vi "main-sequential.vi"() -> ()   [LabVIEW 2024]
uses:
  controls/thermocouple-input-cluster.ctl
  controls/analog-input-cluster.ctl
  controls/analog-output-cluster.ctl
  controls/digitial-input-cluster.ctl
  controls/digital-output-cluster.ctl
  controls/adam-module-select-tab.ctl
  controls/adam-5000-serial-settings.ctl
  controls/state-enum.ctl
  controls/adam-5000-all-chassis-data.ctl
  controls/adam-5000-all-module-datas.ctl
  controls/adam-5000-chassis-cmd-ack.ctl
  controls/adam-5000-module-cmd-ack.ctl
  <vilib>/Instr/_visa.llb/VISA Configure Serial Port (Instr).vi
  <vilib>/Instr/_visa.llb/VISA Flush IO Buffer Mask.ctl
panel:
  out "response":string
  out "cmd string":string
  out "Ack":bool
  out "Sampling":bool
  in  "Slot 1: Module Type":T1(ring)=enum."Thermocouple"
  out "slot: 1":T2
  in  "Digital Outputs 2":T3
  out "Digital Inputs 2":T4
  in  "Analog Outputs 2":T5
  out "Analog Inputs 2":T6
  out "Thermocouple Inputs (degC) 2":T7
  out "response":string
  out "cmd string":string
  out "Ack":bool
  out "Sampling":bool
  in  "Slot 0: Module Type":T1(ring)=enum."Analog Input"
  out "slot: 0":T2
  in  "Digital Outputs":T3
  out "Digital Inputs":T4
  in  "Analog Outputs":T5
  out "Analog Inputs":T6
  out "Thermocouple Inputs (degC)":T7
  in  "Chassis Settings":T8={"VISA resource name"="COM10", "baud rate (19200)"=19200, "Chassis ID"=1}
  in  "Debug Mode":bool
  out "Loop Time (mS)":u32
  out "Loop Counter":i32
  out "Write Success":bool
  out "error IO":errorcluster
  out "error":errorcluster
  in  "exit":bool
  # "ADAM 5000 Controller"
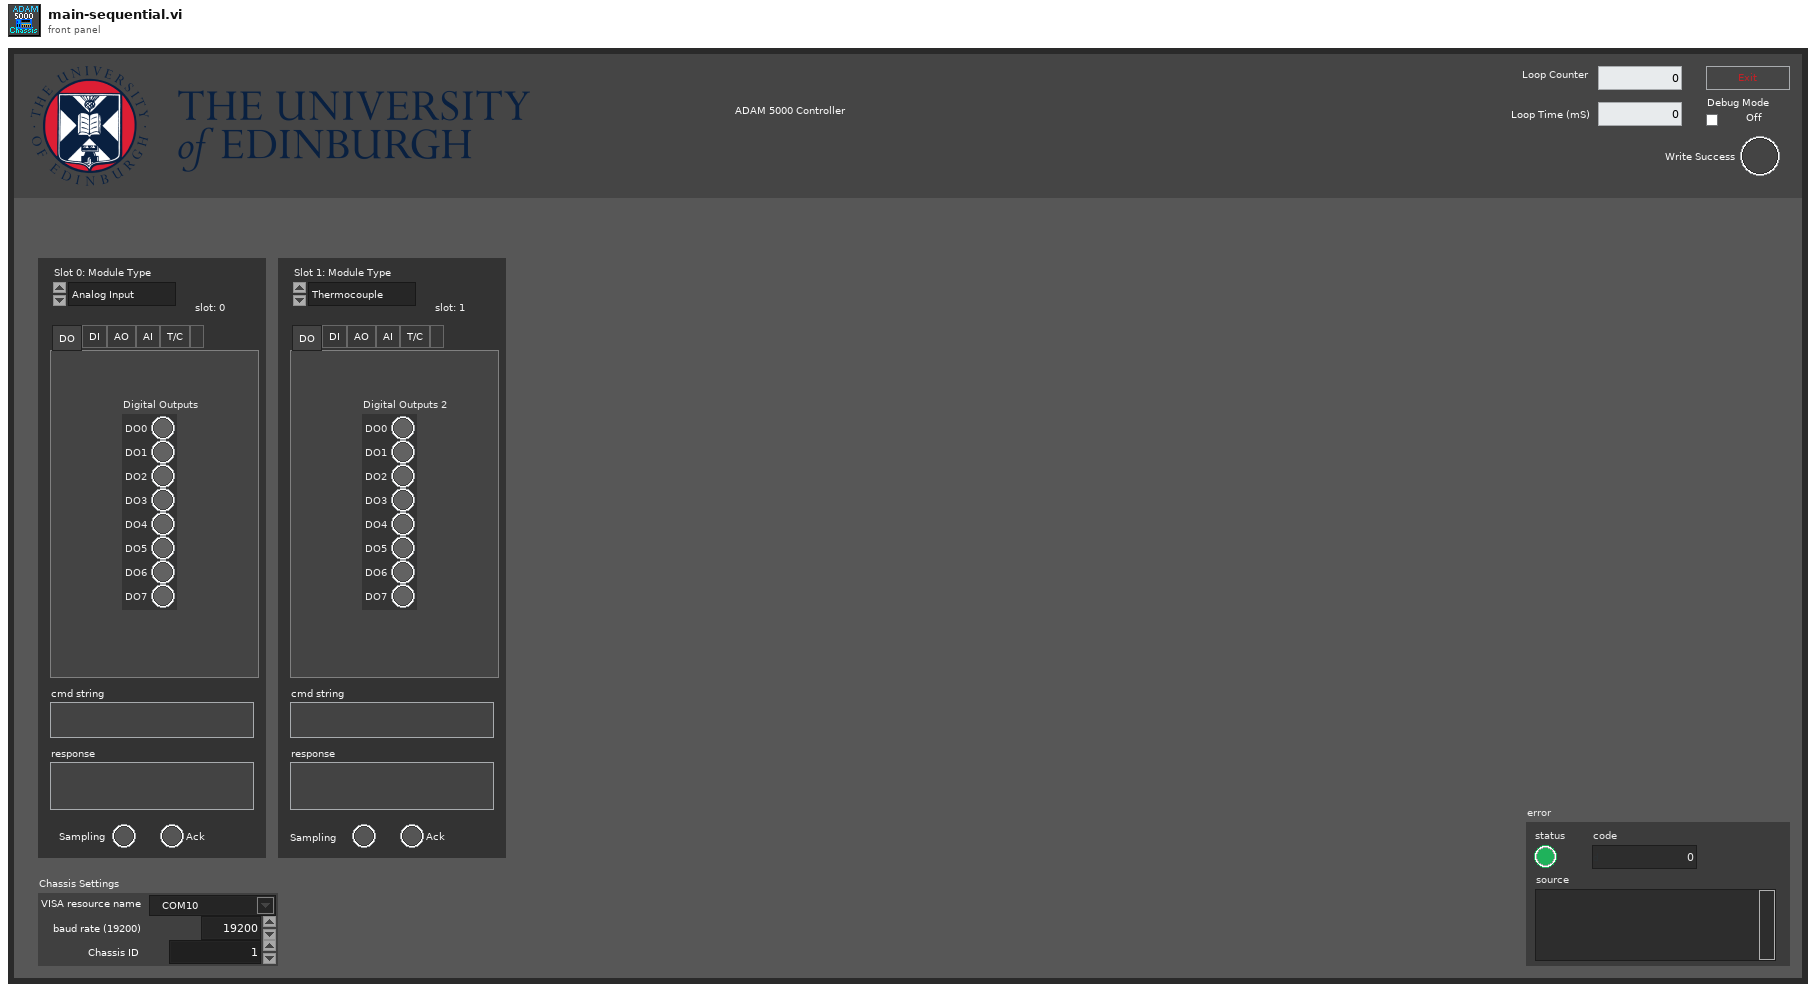
[diagram p1: front panel]
types:
  T1 = enum16{"Digital Output", "Digital Input", "Analog Output", "Analog Input", "Thermocouple", "Power Relay", "empty"}
  T2 = typedef "adam-module-select-tab.ctl" = enum32{"DO", "DI", "AO", "AI", "T/C", ""}
  T3 = typedef "digital-output-cluster.ctl" = cluster{"DO0":bool, "DO1":bool, "DO2":bool, "DO3":bool, "DO4":bool, "DO5":bool, "DO6":bool, "DO7":bool}
  T4 = typedef "digitial-input-cluster.ctl" = cluster{"DI0":bool, "DI1":bool, "DI2":bool, "DI3":bool, "DI4":bool, "DI5":bool, "DI6":bool, "DI7":bool}
  T5 = typedef "analog-output-cluster.ctl" = cluster{"AO0":dbl, "AO1":dbl, "AO2":dbl, "AO3":dbl}
  T6 = typedef "analog-input-cluster.ctl" = cluster{"AI0":dbl, "AI1":dbl, "AI2":dbl, "AI3":dbl, "AI4":dbl, "AI5":dbl, "AI6":dbl, "AI7":dbl}
  T7 = typedef "thermocouple-input-cluster.ctl" = cluster{"TC0":dbl, "TC1":dbl, "TC2":dbl, "TC3":dbl, "TC4":dbl, "TC5":dbl, "TC6":dbl}
  T8 = typedef "adam-5000-serial-settings.ctl" = cluster{"VISA resource name":refnum<visa-resource-name>, "baud rate (19200)":u32, "Chassis ID":u8}
  T9 = typedef "adam-5000-chassis-cmd-ack.ctl" = cluster{"0 cmd-ack":T10, "1 cmd-ack":T10, "2 cmd-ack":T10, "3 cmd-ack":T10, "4 cmd-ack":T10, "5 cmd-ack":T10, "6 cmd-ack":T10, "7 cmd-ack":T10}
  T10 = typedef "adam-5000-module-cmd-ack.ctl" = cluster{"cmd out":string, "acknowledge char":string}
  T11 = typedef "adam-5000-all-chassis-data.ctl" = cluster{"slot:0":T12, "slot:1":T12, "slot:2":T12, "slot:3":T12, "slot:4":T12, "slot:5":T12, "slot:6":T12, "slot:7":T12}
  T12 = typedef "adam-5000-all-module-datas.ctl" = cluster{"Digital Outputs":T3, "Digital Inputs":T4, "Analog Outputs":T5, "Analog Inputs":T6, "Thermocouple Inputs (degC)":T7}
  T13 = typedef "state-enum.ctl" = enum16{"init", "manual", "start", "run", "hold", "stop", ""}
  T14 = cluster{"Analog Outputs":T5, "Analog Outputs 2":T5}
  T15 = cluster{"Slot 0: Module Type":enum16{"Digital Output", "Digital Input", "Analog Output", "Analog Input", "Thermocouple", "Power Relay", "empty"}, "Slot 1: Module Type":enum16{"Digital Output", "Digital Input", "Analog Output", "Analog Input", "Thermocouple", "Power Relay", "empty"}}
  T16 = cluster{"Digital Outputs":T3, "Digital Outputs 2":T3}
  T17 = cluster{"[0]":T10, "[1]":T10, "[2]":T10, "[3]":T10, "[4]":T10, "[5]":T10, "[6]":T10, "[7]":T10, "[8]":T10}
  T18 = typedef "VISA Flush IO Buffer Mask.ctl" = u16
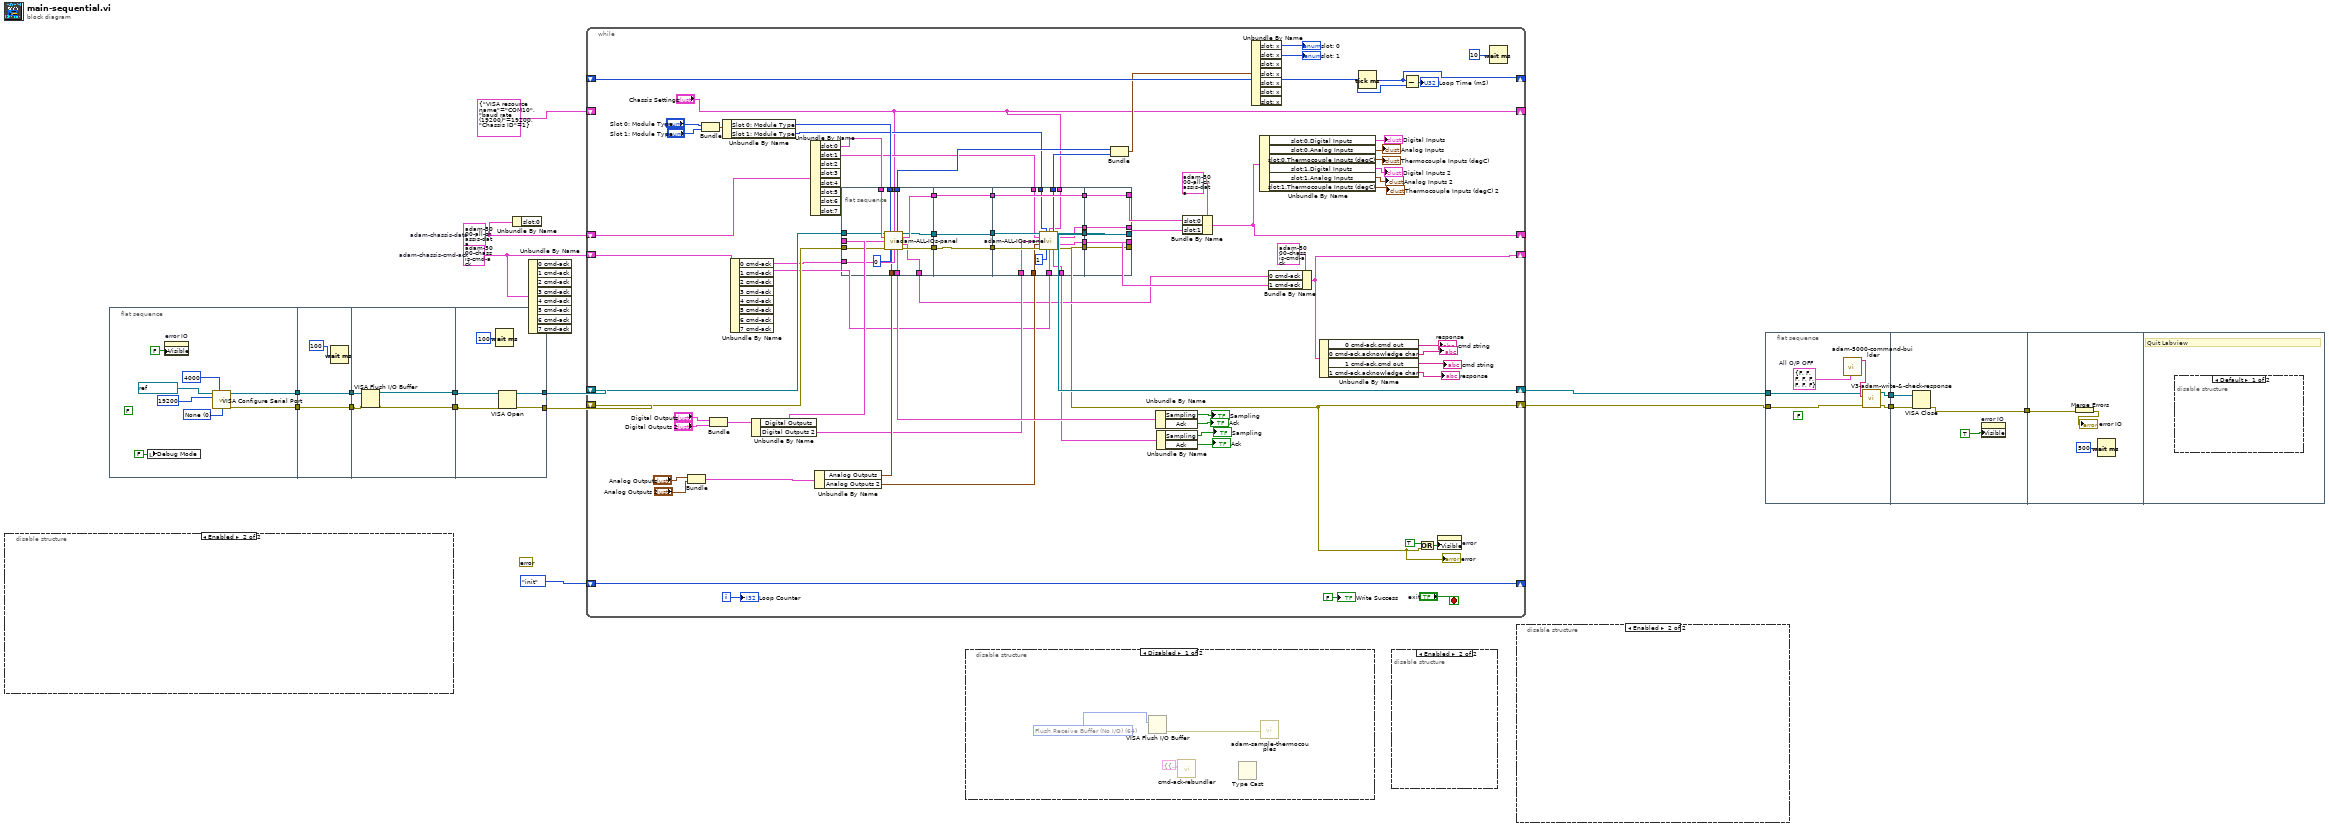
[diagram p0: block diagram]
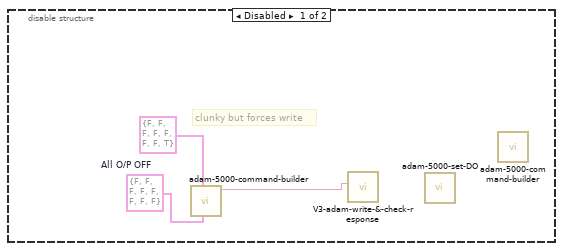
[diagram p2: hidden frame]
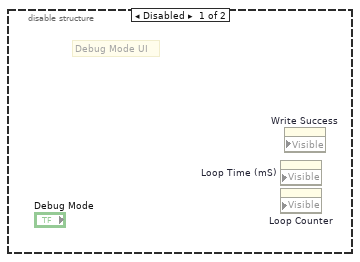
[diagram p3: hidden frame]
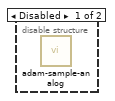
[diagram p4: hidden frame]
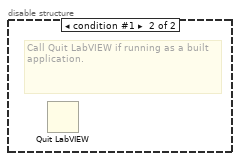
[diagram p6: hidden frame]
diagram:
  w1 = T9 {"0 cmd-ack"={"cmd out"="", "acknowledge char"=""}, "1 cmd-ack"={"cmd out"="", "acknowledge char"=""}, "2 cmd-ack"={"cmd out"="", "acknowledge char"=""}, "3 cmd-ack"={"cmd out"="", "acknowledge char"=""}, "4 cmd-ack"={"cmd out"="", "acknowledge char"=""}, "5 cmd-ack"={"cmd out"="", "acknowledge char"=""}, "6 cmd-ack"={"cmd out"="", "acknowledge char"=""}, "7 cmd-ack"={"cmd out"="", "acknowledge char"=""}}  # adam-chassis-cmd-ack
  w2 = T11 {"slot:0"={"Digital Outputs"={"DO0"=FALSE, "DO1"=FALSE, "DO2"=FALSE, "DO3"=FALSE, "DO4"=FALSE, "DO5"=FALSE, "DO6"=FALSE, "DO7"=FALSE}, "Digital Inputs"={"DI0"=FALSE, "DI1"=FALSE, "DI2"=FALSE, "DI3"=FALSE, "DI4"=FALSE, "DI5"=FALSE, "DI6"=FALSE, "DI7"=FALSE}, "Analog Outputs"={"AO0"=0.0, "AO1"=0.0, "AO2"=0.0, "AO3"=0.0}, "Analog Inputs"={"AI0"=0.0, "AI1"=0.0, "AI2"=0.0, "AI3"=0.0, "AI4"=0.0, "AI5"=0.0, "AI6"=0.0, "AI7"=0.0}, "Thermocouple Inputs (degC)"={"TC0"=0.0, "TC1"=0.0, "TC2"=0.0, "TC3"=0.0, "TC4"=0.0, "TC5"=0.0, "TC6"=0.0}}, "slot:1"={"Digital Outputs"={"DO0"=FALSE, "DO1"=FALSE, "DO2"=FALSE, "DO3"=FALSE, "DO4"=FALSE, "DO5"=FALSE, "DO6"=FALSE, "DO7"=FALSE}, "Digital Inputs"={"DI0"=FALSE, "DI1"=FALSE, "DI2"=FALSE, "DI3"=FALSE, "DI4"=FALSE, "DI5"=FALSE, "DI6"=FALSE, "DI7"=FALSE}, "Analog Outputs"={"AO0"=0.0, "AO1"=0.0, "AO2"=0.0, "AO3"=0.0}, "Analog Inputs"={"AI0"=0.0, "AI1"=0.0, "AI2"=0.0, "AI3"=0.0, "AI4"=0.0, "AI5"=0.0, "AI6"=0.0, "AI7"=0.0}, "Thermocouple Inputs (degC)"={"TC0"=0.0, "TC1"=0.0, "TC2"=0.0, "TC3"=0.0, "TC4"=0.0, "TC5"=0.0, "TC6"=0.0}}, "slot:2"={"Digital Outputs"={"DO0"=FALSE, "DO1"=FALSE, "DO2"=FALSE, "DO3"=FALSE, "DO4"=FALSE, "DO5"=FALSE, "DO6"=FALSE, "DO7"=FALSE}, "Digital Inputs"={"DI0"=FALSE, "DI1"=FALSE, "DI2"=FALSE, "DI3"=FALSE, "DI4"=FALSE, "DI5"=FALSE, "DI6"=FALSE, "DI7"=FALSE}, "Analog Outputs"={"AO0"=0.0, "AO1"=0.0, "AO2"=0.0, "AO3"=0.0}, "Analog Inputs"={"AI0"=0.0, "AI1"=0.0, "AI2"=0.0, "AI3"=0.0, "AI4"=0.0, "AI5"=0.0, "AI6"=0.0, "AI7"=0.0}, "Thermocouple Inputs (degC)"={"TC0"=0.0, "TC1"=0.0, "TC2"=0.0, "TC3"=0.0, "TC4"=0.0, "TC5"=0.0, "TC6"=0.0}}, "slot:3"={"Digital Outputs"={"DO0"=FALSE, "DO1"=FALSE, "DO2"=FALSE, "DO3"=FALSE, "DO4"=FALSE, "DO5"=FALSE, "DO6"=FALSE, "DO7"=FALSE}, "Digital Inputs"={"DI0"=FALSE, "DI1"=FALSE, "DI2"=FALSE, "DI3"=FALSE, "DI4"=FALSE, "DI5"=FALSE, "DI6"=FALSE, "DI7"=FALSE}, "Analog Outputs"={"AO0"=0.0, "AO1"=0.0, "AO2"=0.0, "AO3"=0.0}, "Analog Inputs"={"AI0"=0.0, "AI1"=0.0, "AI2"=0.0, "AI3"=0.0, "AI4"=0.0, "AI5"=0.0, "AI6"=0.0, "AI7"=0.0}, "Thermocouple Inputs (degC)"={"TC0"=0.0, "TC1"=0.0, "TC2"=0.0, "TC3"=0.0, "TC4"=0.0, "TC5"=0.0, "TC6"=0.0}}, "slot:4"={"Digital Outputs"={"DO0"=FALSE, "DO1"=FALSE, "DO2"=FALSE, "DO3"=FALSE, "DO4"=FALSE, "DO5"=FALSE, "DO6"=FALSE, "DO7"=FALSE}, "Digital Inputs"={"DI0"=FALSE, "DI1"=FALSE, "DI2"=FALSE, "DI3"=FALSE, "DI4"=FALSE, "DI5"=FALSE, "DI6"=FALSE, "DI7"=FALSE}, "Analog Outputs"={"AO0"=0.0, "AO1"=0.0, "AO2"=0.0, "AO3"=0.0}, "Analog Inputs"={"AI0"=0.0, "AI1"=0.0, "AI2"=0.0, "AI3"=0.0, "AI4"=0.0, "AI5"=0.0, "AI6"=0.0, "AI7"=0.0}, "Thermocouple Inputs (degC)"={"TC0"=0.0, "TC1"=0.0, "TC2"=0.0, "TC3"=0.0, "TC4"=0.0, "TC5"=0.0, "TC6"=0.0}}, "slot:5"={"Digital Outputs"={"DO0"=FALSE, "DO1"=FALSE, "DO2"=FALSE, "DO3"=FALSE, "DO4"=FALSE, "DO5"=FALSE, "DO6"=FALSE, "DO7"=FALSE}, "Digital Inputs"={"DI0"=FALSE, "DI1"=FALSE, "DI2"=FALSE, "DI3"=FALSE, "DI4"=FALSE, "DI5"=FALSE, "DI6"=FALSE, "DI7"=FALSE}, "Analog Outputs"={"AO0"=0.0, "AO1"=0.0, "AO2"=0.0, "AO3"=0.0}, "Analog Inputs"={"AI0"=0.0, "AI1"=0.0, "AI2"=0.0, "AI3"=0.0, "AI4"=0.0, "AI5"=0.0, "AI6"=0.0, "AI7"=0.0}, "Thermocouple Inputs (degC)"={"TC0"=0.0, "TC1"=0.0, "TC2"=0.0, "TC3"=0.0, "TC4"=0.0, "TC5"=0.0, "TC6"=0.0}}, "slot:6"={"Digital Outputs"={"DO0"=FALSE, "DO1"=FALSE, "DO2"=FALSE, "DO3"=FALSE, "DO4"=FALSE, "DO5"=FALSE, "DO6"=FALSE, "DO7"=FALSE}, "Digital Inputs"={"DI0"=FALSE, "DI1"=FALSE, "DI2"=FALSE, "DI3"=FALSE, "DI4"=FALSE, "DI5"=FALSE, "DI6"=FALSE, "DI7"=FALSE}, "Analog Outputs"={"AO0"=0.0, "AO1"=0.0, "AO2"=0.0, "AO3"=0.0}, "Analog Inputs"={"AI0"=0.0, "AI1"=0.0, "AI2"=0.0, "AI3"=0.0, "AI4"=0.0, "AI5"=0.0, "AI6"=0.0, "AI7"=0.0}, "Thermocouple Inputs (degC)"={"TC0"=0.0, "TC1"=0.0, "TC2"=0.0, "TC3"=0.0, "TC4"=0.0, "TC5"=0.0, "TC6"=0.0}}, "slot:7"={"Digital Outputs"={"DO0"=FALSE, "DO1"=FALSE, "DO2"=FALSE, "DO3"=FALSE, "DO4"=FALSE, "DO5"=FALSE, "DO6"=FALSE, "DO7"=FALSE}, "Digital Inputs"={"DI0"=FALSE, "DI1"=FALSE, "DI2"=FALSE, "DI3"=FALSE, "DI4"=FALSE, "DI5"=FALSE, "DI6"=FALSE, "DI7"=FALSE}, "Analog Outputs"={"AO0"=0.0, "AO1"=0.0, "AO2"=0.0, "AO3"=0.0}, "Analog Inputs"={"AI0"=0.0, "AI1"=0.0, "AI2"=0.0, "AI3"=0.0, "AI4"=0.0, "AI5"=0.0, "AI6"=0.0, "AI7"=0.0}, "Thermocouple Inputs (degC)"={"TC0"=0.0, "TC1"=0.0, "TC2"=0.0, "TC3"=0.0, "TC4"=0.0, "TC5"=0.0, "TC6"=0.0}}}  # adam-chassis-data
  (unwired) errorcluster {"status"=FALSE, "code"=0, "source"=""} ("error")
  n1 = disable-structure shown="Enabled" {
    frame Disabled {
      w20 = T3 {"DO0"=FALSE, "DO1"=FALSE, "DO2"=FALSE, "DO3"=FALSE, "DO4"=FALSE, "DO5"=FALSE, "DO6"=FALSE, "DO7"=FALSE}  # All O/P OFF
      # "clunky but forces write"
      n2 = call "adam-5000-command-builder.vi"("Output Control"=w20, "Current Output State"=T3 {"DO0"=FALSE, "DO1"=FALSE, "DO2"=FALSE, "DO3"=FALSE, "DO4"=FALSE, "DO5"=FALSE, "DO6"=FALSE, "DO7"=TRUE}) -> ("Command Out"=w19:string)  [unwired: 7 in, 2 out]
      n3 = call "V3-adam-write-&-check-response.vi"("write buffer"=w19) -> ("VISA resource name"=w18:refnum<visa-resource-name>)  [unwired: 5 in, 5 out]
      n4 = call "adam-5000-set-DO.vi"() -> ()  [unwired: 6 in, 6 out]
      n5 = call "adam-5000-command-builder.vi"() -> ()  [unwired: 9 in, 3 out]
    }
    frame Enabled {
    }
  }
  n6 = flat-sequence {
    tunnel: [w28] -> w11
    tunnel: [w27] -> w10
    tunnel: w11 -> [w32]
    tunnel: [w32] -> w9
    tunnel: w10 -> [w31]
    tunnel: [w31] -> w8
    tunnel: w9 -> [w36]
    tunnel: [w34] -> w7
    tunnel: w8 -> [w35]
    tunnel: [w33] -> w6
    tunnel: w7 -> [w40]
    tunnel: w6 -> [w39]
    tunnel: [w38] -> w5
    tunnel: [w37] -> w4
    frame #0 {
      w25 = u16 0 items=["None", "XON/XOFF", "RTS/CTS", "XON/XOFF & RTS/CTS", "DTR/DSR", "XON/XOFF & DTR/DSR"] ("flow control (0:none)")
      (unwired) FALSE ("V1")
      n7 = local write "Debug Mode"(FALSE ("Debug Mode")) -> ()
      n8 = property on="error IO" class="Clust (strict)"("Visible"=FALSE) -> ()  [unwired: 2 in, 2 out]
      n9 = call-poly "VISA Configure Serial Port"("VISA resource name"=refnum<visa-resource-name> "COM10", "timeout (10sec)"=u32 4000, "baud rate (9600)"=u32 19200, "flow control (0:none)"=w25) -> ("VISA resource name out"=w28:refnum<visa-resource-name>, "error out"=w27:errorcluster)  [unwired: 10 in]
    }
    frame #1 {
      n10 = Wait (ms)(milliseconds to wait=u32 100) -> ()  [unwired: 1 out]
    }
    frame #2 {
      n11 = VISA Flush I/O Buffer(VISA resource name=w36, error in (no error)=w35) -> (VISA resource name out=w34:refnum<visa-resource-name>, error out=w33:errorcluster)  [unwired: 1 in]
    }
    frame #3 {
      n12 = Wait (ms)(milliseconds to wait=u32 100) -> ()  [unwired: 1 out]
      n13 = VISA Open(error in (no error)=w39, VISA resource name=w40) -> (VISA resource name=w38:refnum<visa-resource-name>, error out=w37:errorcluster)  [unwired: 3 in]
    }
  }
  n14 = Unbundle By Name(w2) -> ()  [unwired: 1 out]
  n15 = Unbundle By Name(w1) -> ()  [unwired: 8 out]
  n16 = while {
    shift-right: [w109] -> _
    shift-left: state-enum."init" ("state-enum") -> [w109]
    shift-right: [w48] -> w16
    shift-left: w4 -> [w90]
    shift-right: [w112] -> _
    shift-left: _ -> [w114]
    shift-right: ["Chassis Settings"] -> _
    shift-left: T8 {"VISA resource name"="COM10", "baud rate (19200)"=19200, "Chassis ID"=1} ("Chassis Settings") -> [_]
    shift-right: [w69] -> w3
    shift-left: w5 -> [w91]
    shift-right: [w74] -> _
    shift-left: w2 -> [w42]
    shift-right: [w85] -> _
    shift-left: w1 -> [w93]
    i -> [w115]
    stop <- "exit" stop-if-true
    n17 = Bundle("Analog Outputs"="Analog Outputs", "Analog Outputs 2"="Analog Outputs 2") -> (w82:T14)  [unwired: 1 in]
    n18 = Bundle("Slot 0: Module Type"="Slot 0: Module Type", "Slot 1: Module Type"="Slot 1: Module Type") -> (w80:T15)  [unwired: 1 in]
    n19 = Bundle("Digital Outputs"="Digital Outputs", "Digital Outputs 2"="Digital Outputs 2") -> (w84:T16)  [unwired: 1 in]
    n20 = Unbundle By Name(w80) -> ("Slot 0: Module Type"=w79:T1, "Slot 1: Module Type"=w59:T1)
    n21 = Unbundle By Name(w93) -> ("0 cmd-ack"=w89:T10, "1 cmd-ack"=w61:T10)  [unwired: 6 out]
    n22 = Unbundle By Name(w84) -> ("Digital Outputs"=w83:T3, "Digital Outputs 2"=w63:T3)
    n23 = Unbundle By Name(w42) -> ("slot:0"=w92:T12, "slot:1"=w65:T12)  [unwired: 6 out]
    n24 = Unbundle By Name(w82) -> ("Analog Outputs"=w81:T5, "Analog Outputs 2"=w62:T5)
    n25 = flat-sequence {
      tunnel: w92 -> [w132]
      tunnel: w91 -> [w131]
      tunnel: w90 -> [w130]
      tunnel: w89 -> [w129]
      tunnel: w83 -> [w127]
      tunnel: w81 -> [w126]
      tunnel: "Chassis Settings" -> [w125]
      tunnel: w79 -> [w124]
      tunnel: [w123] -> w78
      tunnel: [w121] -> w68
      tunnel: [w128] -> w55
      tunnel: [w122] -> w53
      tunnel: [w119] -> w51
      tunnel: [w118] -> w49
      tunnel: w55 -> [w135]
      tunnel: [w135] -> w54
      tunnel: w53 -> [w134]
      tunnel: [w134] -> w52
      tunnel: w51 -> [w133]
      tunnel: [w133] -> w50
      tunnel: w54 -> [w151]
      tunnel: w52 -> [w150]
      tunnel: w50 -> [w148]
      tunnel: w65 -> [w146]
      tunnel: w63 -> [w144]
      tunnel: w62 -> [w143]
      tunnel: w61 -> [w141]
      tunnel: w59 -> [w139]
      tunnel: [w138] -> w58
      tunnel: "Chassis Settings" -> [w137]
      tunnel: [w136] -> w56
      tunnel: [w151] -> w47
      tunnel: [w149] -> w46
      tunnel: [w147] -> w45
      tunnel: [w145] -> w44
      tunnel: [w140] -> w43
      tunnel: [w152] -> w60
      tunnel: [w153] -> w64
      tunnel: [w154] -> w48
      tunnel: [w155] -> w69
      tunnel: [w156] -> w87
      tunnel: w47 -> [w156]
      tunnel: w46 -> [w155]
      tunnel: w45 -> [w154]
      tunnel: w44 -> [w153]
      tunnel: w43 -> [w152]
      frame #0 {
        n26 = call "adam-ALL-IOs-panel.vi"("VISA Refnum in"=w131, "Module Type"=w124, "Chassis Settings"=w125, "ADAM-5000-data-current"=w132, "Digital Outputs"=w127, "Analog Outputs"=w126, "error in (no error)"=w130, "chassis-slot"=0, "cmd-ack-in"=w129) -> ("slot: x"=w123:T2, "VISA Refnum out"=w122:refnum<visa-resource-name>, "ADAM-5000-data-new"=w128:T12, "cmd-ack-out"=w118:T10, "status-cluster"=w121:cluster{"Sampling":bool, "Ack":bool}, "error out"=w119:errorcluster)  [unwired: 1 in]
      }
      frame #1 {
      }
      frame #2 {
        n27 = call "adam-ALL-IOs-panel.vi"("VISA Refnum in"=w150, "Module Type"=w139, "Chassis Settings"=w137, "ADAM-5000-data-current"=w146, "Digital Outputs"=w144, "Analog Outputs"=w143, "error in (no error)"=w148, "chassis-slot"=1, "cmd-ack-in"=w141) -> ("slot: x"=w138:T2, "VISA Refnum out"=w149:refnum<visa-resource-name>, "ADAM-5000-data-new"=w145:T12, "cmd-ack-out"=w140:T10, "status-cluster"=w136:cluster{"Sampling":bool, "Ack":bool}, "error out"=w147:errorcluster)  [unwired: 1 in]
      }
      frame #3 {
      }
    }
    n28 = Bundle("slot: x"=w78, "slot: x"=w58) -> (w77:cluster{"slot: x":T2, "slot: x":T2})  [unwired: 1 in]
    n29 = Unbundle By Name(w68) -> ("Sampling"=→"Sampling":bool, "Ack"=→"Ack":bool)
    n30 = Unbundle By Name(w56) -> ("Sampling"=→"Sampling":bool, "Ack"=→"Ack":bool)
    n31 = Bundle By Name(cluster=T11 {"slot:0"={"Digital Outputs"={"DO0"=FALSE, "DO1"=FALSE, "DO2"=FALSE, "DO3"=FALSE, "DO4"=FALSE, "DO5"=FALSE, "DO6"=FALSE, "DO7"=FALSE}, "Digital Inputs"={"DI0"=FALSE, "DI1"=FALSE, "DI2"=FALSE, "DI3"=FALSE, "DI4"=FALSE, "DI5"=FALSE, "DI6"=FALSE, "DI7"=FALSE}, "Analog Outputs"={"AO0"=0.0, "AO1"=0.0, "AO2"=0.0, "AO3"=0.0}, "Analog Inputs"={"AI0"=0.0, "AI1"=0.0, "AI2"=0.0, "AI3"=0.0, "AI4"=0.0, "AI5"=0.0, "AI6"=0.0, "AI7"=0.0}, "Thermocouple Inputs (degC)"={"TC0"=0.0, "TC1"=0.0, "TC2"=0.0, "TC3"=0.0, "TC4"=0.0, "TC5"=0.0, "TC6"=0.0}}, "slot:1"={"Digital Outputs"={"DO0"=FALSE, "DO1"=FALSE, "DO2"=FALSE, "DO3"=FALSE, "DO4"=FALSE, "DO5"=FALSE, "DO6"=FALSE, "DO7"=FALSE}, "Digital Inputs"={"DI0"=FALSE, "DI1"=FALSE, "DI2"=FALSE, "DI3"=FALSE, "DI4"=FALSE, "DI5"=FALSE, "DI6"=FALSE, "DI7"=FALSE}, "Analog Outputs"={"AO0"=0.0, "AO1"=0.0, "AO2"=0.0, "AO3"=0.0}, "Analog Inputs"={"AI0"=0.0, "AI1"=0.0, "AI2"=0.0, "AI3"=0.0, "AI4"=0.0, "AI5"=0.0, "AI6"=0.0, "AI7"=0.0}, "Thermocouple Inputs (degC)"={"TC0"=0.0, "TC1"=0.0, "TC2"=0.0, "TC3"=0.0, "TC4"=0.0, "TC5"=0.0, "TC6"=0.0}}, "slot:2"={"Digital Outputs"={"DO0"=FALSE, "DO1"=FALSE, "DO2"=FALSE, "DO3"=FALSE, "DO4"=FALSE, "DO5"=FALSE, "DO6"=FALSE, "DO7"=FALSE}, "Digital Inputs"={"DI0"=FALSE, "DI1"=FALSE, "DI2"=FALSE, "DI3"=FALSE, "DI4"=FALSE, "DI5"=FALSE, "DI6"=FALSE, "DI7"=FALSE}, "Analog Outputs"={"AO0"=0.0, "AO1"=0.0, "AO2"=0.0, "AO3"=0.0}, "Analog Inputs"={"AI0"=0.0, "AI1"=0.0, "AI2"=0.0, "AI3"=0.0, "AI4"=0.0, "AI5"=0.0, "AI6"=0.0, "AI7"=0.0}, "Thermocouple Inputs (degC)"={"TC0"=0.0, "TC1"=0.0, "TC2"=0.0, "TC3"=0.0, "TC4"=0.0, "TC5"=0.0, "TC6"=0.0}}, "slot:3"={"Digital Outputs"={"DO0"=FALSE, "DO1"=FALSE, "DO2"=FALSE, "DO3"=FALSE, "DO4"=FALSE, "DO5"=FALSE, "DO6"=FALSE, "DO7"=FALSE}, "Digital Inputs"={"DI0"=FALSE, "DI1"=FALSE, "DI2"=FALSE, "DI3"=FALSE, "DI4"=FALSE, "DI5"=FALSE, "DI6"=FALSE, "DI7"=FALSE}, "Analog Outputs"={"AO0"=0.0, "AO1"=0.0, "AO2"=0.0, "AO3"=0.0}, "Analog Inputs"={"AI0"=0.0, "AI1"=0.0, "AI2"=0.0, "AI3"=0.0, "AI4"=0.0, "AI5"=0.0, "AI6"=0.0, "AI7"=0.0}, "Thermocouple Inputs (degC)"={"TC0"=0.0, "TC1"=0.0, "TC2"=0.0, "TC3"=0.0, "TC4"=0.0, "TC5"=0.0, "TC6"=0.0}}, "slot:4"={"Digital Outputs"={"DO0"=FALSE, "DO1"=FALSE, "DO2"=FALSE, "DO3"=FALSE, "DO4"=FALSE, "DO5"=FALSE, "DO6"=FALSE, "DO7"=FALSE}, "Digital Inputs"={"DI0"=FALSE, "DI1"=FALSE, "DI2"=FALSE, "DI3"=FALSE, "DI4"=FALSE, "DI5"=FALSE, "DI6"=FALSE, "DI7"=FALSE}, "Analog Outputs"={"AO0"=0.0, "AO1"=0.0, "AO2"=0.0, "AO3"=0.0}, "Analog Inputs"={"AI0"=0.0, "AI1"=0.0, "AI2"=0.0, "AI3"=0.0, "AI4"=0.0, "AI5"=0.0, "AI6"=0.0, "AI7"=0.0}, "Thermocouple Inputs (degC)"={"TC0"=0.0, "TC1"=0.0, "TC2"=0.0, "TC3"=0.0, "TC4"=0.0, "TC5"=0.0, "TC6"=0.0}}, "slot:5"={"Digital Outputs"={"DO0"=FALSE, "DO1"=FALSE, "DO2"=FALSE, "DO3"=FALSE, "DO4"=FALSE, "DO5"=FALSE, "DO6"=FALSE, "DO7"=FALSE}, "Digital Inputs"={"DI0"=FALSE, "DI1"=FALSE, "DI2"=FALSE, "DI3"=FALSE, "DI4"=FALSE, "DI5"=FALSE, "DI6"=FALSE, "DI7"=FALSE}, "Analog Outputs"={"AO0"=0.0, "AO1"=0.0, "AO2"=0.0, "AO3"=0.0}, "Analog Inputs"={"AI0"=0.0, "AI1"=0.0, "AI2"=0.0, "AI3"=0.0, "AI4"=0.0, "AI5"=0.0, "AI6"=0.0, "AI7"=0.0}, "Thermocouple Inputs (degC)"={"TC0"=0.0, "TC1"=0.0, "TC2"=0.0, "TC3"=0.0, "TC4"=0.0, "TC5"=0.0, "TC6"=0.0}}, "slot:6"={"Digital Outputs"={"DO0"=FALSE, "DO1"=FALSE, "DO2"=FALSE, "DO3"=FALSE, "DO4"=FALSE, "DO5"=FALSE, "DO6"=FALSE, "DO7"=FALSE}, "Digital Inputs"={"DI0"=FALSE, "DI1"=FALSE, "DI2"=FALSE, "DI3"=FALSE, "DI4"=FALSE, "DI5"=FALSE, "DI6"=FALSE, "DI7"=FALSE}, "Analog Outputs"={"AO0"=0.0, "AO1"=0.0, "AO2"=0.0, "AO3"=0.0}, "Analog Inputs"={"AI0"=0.0, "AI1"=0.0, "AI2"=0.0, "AI3"=0.0, "AI4"=0.0, "AI5"=0.0, "AI6"=0.0, "AI7"=0.0}, "Thermocouple Inputs (degC)"={"TC0"=0.0, "TC1"=0.0, "TC2"=0.0, "TC3"=0.0, "TC4"=0.0, "TC5"=0.0, "TC6"=0.0}}, "slot:7"={"Digital Outputs"={"DO0"=FALSE, "DO1"=FALSE, "DO2"=FALSE, "DO3"=FALSE, "DO4"=FALSE, "DO5"=FALSE, "DO6"=FALSE, "DO7"=FALSE}, "Digital Inputs"={"DI0"=FALSE, "DI1"=FALSE, "DI2"=FALSE, "DI3"=FALSE, "DI4"=FALSE, "DI5"=FALSE, "DI6"=FALSE, "DI7"=FALSE}, "Analog Outputs"={"AO0"=0.0, "AO1"=0.0, "AO2"=0.0, "AO3"=0.0}, "Analog Inputs"={"AI0"=0.0, "AI1"=0.0, "AI2"=0.0, "AI3"=0.0, "AI4"=0.0, "AI5"=0.0, "AI6"=0.0, "AI7"=0.0}, "Thermocouple Inputs (degC)"={"TC0"=0.0, "TC1"=0.0, "TC2"=0.0, "TC3"=0.0, "TC4"=0.0, "TC5"=0.0, "TC6"=0.0}}}, "slot:0"=w87, "slot:1"=w64) -> (w74:T11)
    n32 = Unbundle By Name(w77) -> ("slot: x"=→"slot: 0":T2, "slot: x"=→"slot: 1":T2)  [unwired: 5 out]
    n33 = Unbundle By Name(w74) -> ("slot:0.Digital Inputs"=→"Digital Inputs":T4, "slot:0.Analog Inputs"=→"Analog Inputs":T6, "slot:0.Thermocouple Inputs (degC)"=→"Thermocouple Inputs (degC)":T7, "slot:1.Digital Inputs"=→"Digital Inputs 2":T4, "slot:1.Analog Inputs"=→"Analog Inputs 2":T6, "slot:1.Thermocouple Inputs (degC)"=→"Thermocouple Inputs (degC) 2":T7)
    n34 = Bundle By Name(cluster=T9 {"0 cmd-ack"={"cmd out"="", "acknowledge char"=""}, "1 cmd-ack"={"cmd out"="", "acknowledge char"=""}, "2 cmd-ack"={"cmd out"="", "acknowledge char"=""}, "3 cmd-ack"={"cmd out"="", "acknowledge char"=""}, "4 cmd-ack"={"cmd out"="", "acknowledge char"=""}, "5 cmd-ack"={"cmd out"="", "acknowledge char"=""}, "6 cmd-ack"={"cmd out"="", "acknowledge char"=""}, "7 cmd-ack"={"cmd out"="", "acknowledge char"=""}} ("adam-chassis-cmd-ack"), "0 cmd-ack"=w49, "1 cmd-ack"=w60) -> (w85:T9)
    n35 = Unbundle By Name(w85) -> ("0 cmd-ack.cmd out"=→"cmd string":string, "0 cmd-ack.acknowledge char"=→"response":string, "1 cmd-ack.cmd out"=→"cmd string":string, "1 cmd-ack.acknowledge char"=→"response":string)
    n36 = Tick Count (ms)() -> (millisecond timer value=w112:u32)
    n37 = Subtract(x=w112, y=w114) -> (x-y=→"Loop Time (mS)":u32)
    n38 = Or(x=TRUE ("Debug Mode"), y=w48) -> (x .or. y?=w111:bool)
    n39 = property on="error" class="Clust (strict)"("Visible"=w111) -> ()  [unwired: 2 in, 2 out]
    n40 = Wait (ms)(milliseconds to wait=u32 10) -> ()  [unwired: 1 out]
    "error" <- w48
    "Write Success" <- FALSE ("Write Success")
    "Loop Counter" <- w115
  }
  n41 = disable-structure shown="Disabled" {
    frame Disabled {
      w162 = T18 64 items=["Flush Receive Buffer"=16, "Write Transmit Buffer to Device"=32, "Flush Receive Buffer (No I/O)"=64, "Flush Transmit Buffer"=128] ("Mask")
      n42 = VISA Flush I/O Buffer(mask (16)=w162) -> (error out=w161:errorcluster)  [unwired: 2 in, 1 out]
      n43 = call "cmd-ack-rebundler.vi"("cmd-ack-in"=T17 {"[0]"={"cmd out"="", "acknowledge char"=""}, "[1]"={"cmd out"="", "acknowledge char"=""}, "[2]"={"cmd out"="", "acknowledge char"=""}, "[3]"={"cmd out"="", "acknowledge char"=""}, "[4]"={"cmd out"="", "acknowledge char"=""}, "[5]"={"cmd out"="", "acknowledge char"=""}, "[6]"={"cmd out"="", "acknowledge char"=""}, "[7]"={"cmd out"="", "acknowledge char"=""}, "[8]"={"cmd out"="", "acknowledge char"=""}}) -> ()  [unwired: 10 in, 1 out]
      n44 = Type Cast() -> ()  [unwired: 2 in, 1 out]
      n45 = call "adam-sample-thermocouples.vi"("error in (no error)"=w161) -> ("status"=w159:string, "read buffer"=w158:string, "acknowledge char"=w160:string)  [unwired: 5 in, 3 out]
    }
    frame Enabled {
    }
  }
  n46 = disable-structure shown="Enabled" {
    frame Disabled {
      n47 = call "adam-sample-analog.vi"() -> ()  [unwired: 6 in, 6 out]
    }
    frame Enabled {
    }
  }
  n48 = disable-structure shown="Enabled" {
    frame Disabled {
      # "Debug Mode UI"
      n49 = property on="Loop Time (mS)" class="DigNum (strict)" props=["Visible"]() -> ()  [unwired: 3 in, 2 out]
      n50 = property on="Loop Counter" class="DigNum (strict)" props=["Visible"]() -> ()  [unwired: 3 in, 2 out]
      n51 = property on="Write Success" class="Bool (strict)" props=["Visible"]() -> ()  [unwired: 3 in, 2 out]
    }
    frame Enabled {
    }
  }
  n52 = flat-sequence {
    tunnel: w16 -> [w168]
    tunnel: [w167] -> w14
    tunnel: [w166] -> w13
    tunnel: w3 -> [w164]
    tunnel: [w170] -> w15
    tunnel: w14 -> [w171]
    tunnel: w13 -> [w172]
    tunnel: w15 -> [w174]
    frame #0 {
      (unwired) FALSE ("V1")
      w165 = T3 {"DO0"=FALSE, "DO1"=FALSE, "DO2"=FALSE, "DO3"=FALSE, "DO4"=FALSE, "DO5"=FALSE, "DO6"=FALSE, "DO7"=FALSE}  # All O/P OFF
      n53 = call "adam-5000-command-builder.vi"("Output Control"=w165) -> ("Command Out"=w169:string)  [unwired: 8 in, 2 out]
      n54 = call "V3-adam-write-&-check-response.vi"("error in (no error)"=w168, "write buffer"=w169, "VISA resource name"=w164) -> ("error out"=w166:errorcluster, "VISA resource name out"=w167:refnum<visa-resource-name>)  [unwired: 4 in, 3 out]
    }
    frame #1 {
      n55 = VISA Close(VISA resource name=w171, error in (no error)=w172) -> (error out=w170:errorcluster)
      n56 = property on="error IO" class="Clust (strict)"("Visible"=TRUE) -> ()  [unwired: 2 in, 2 out]
    }
    frame #2 {
      n57 = Merge Errors(w174) -> (→"error IO":errorcluster)
      n58 = Wait (ms)(milliseconds to wait=u32 500) -> ()  [unwired: 1 out]
    }
    frame #3 {
      # "Quit Labview"
      n59 = disable-structure "Conditional Disable Structure" shown="Default" {
        frame condition #0 (active) {
        }
        frame condition #1 {
          # "Call Quit LabVIEW if running as a built application."
          n60 = Quit LabVIEW() -> ()  [unwired: 1 in]
        }
      }
    }
  }
